vi "test.vi"() -> ()   [LabVIEW 2020]
uses:
  DSF Core.lvlibp/Typedefs/DSF Engine Framework Configuration.ctl
  DSF Core.lvlibp/Typedefs/DSF Engine Plugin Configuration.ctl
  DSF Core.lvlibp/Typedefs/Core Plugin Configuration.ctl
  DSF Core.lvlibp/Typedefs/DSF Timing Info.ctl
  DSF Core.lvlibp/Typedefs/DSF Settings Info.ctl
  DSF Core.lvlibp/Typedefs/DSF Engine Plugin Thread Configuration.ctl
  DSF Core.lvlibp/Typedefs/Core Thread Configuration.ctl
  DSF Core.lvlibp/Typedefs/DSF Engine Transfer Group Configuration.ctl
  DSF Core.lvlibp/Typedefs/Core Group Configuration.ctl
  DSF Core.lvlibp/Typedefs/DSF Direction.ctl
  DSF Core.lvlibp/Typedefs/DSF Timeout Behavior.ctl
  DSF Core.lvlibp/Typedefs/DSF Engine Transfer Configuration.ctl
  DSF Core.lvlibp/Typedefs/Core Transfer Configuration.ctl
  DSF Core.lvlibp/Typedefs/DSF Engine Channel Configuration.ctl
  DSF Core.lvlibp/Typedefs/Core Channel Configuration.ctl
  DSF Core.lvlibp/Typedefs/DSF Data Type.ctl
  niveristand-data-sharing-framework-custom-device/Source/Core/Built/Configuration API/Component/Default Buffer Converter/Default Buffer Converter Transfer Settings.ctl
  DSF Core.lvlibp/Typedefs/DSF Byte Order.ctl
  Types/Tx Configuration.ctl
  Built/Plugins/Windows/Components/UDP.lvlibp/Configuration/Thread/Thread Settings.ctl
  niveristand-data-sharing-framework-custom-device/Source/Core/Built/Configuration API/DSF Configuration API.lvlib
  DSF Core.lvlibp
  DSF Core.lvlibp/Classes/Configuration/Core/Plugin/Plugin Configuration.lvclass
  DSF Core.lvlibp/Classes/Configuration/Core/Channel/Channel Configuration.lvclass
  DSF Core.lvlibp/Classes/Configuration/Core/Group/Group Configuration.lvclass
  DSF Core.lvlibp/Classes/Configuration/Core/Thread/Thread Configuration.lvclass
  DSF UDP Configuration API.lvlib
  Built/Plugins/Windows/Components/UDP.lvlibp/Configuration/Thread/UDP Thread Configuration.lvclass
  DSF Core.lvlibp/Classes/Configuration/Core/Transfer/Transfer Configuration.lvclass
panel:
  out "framework out":T1
  out "error out":errorcluster
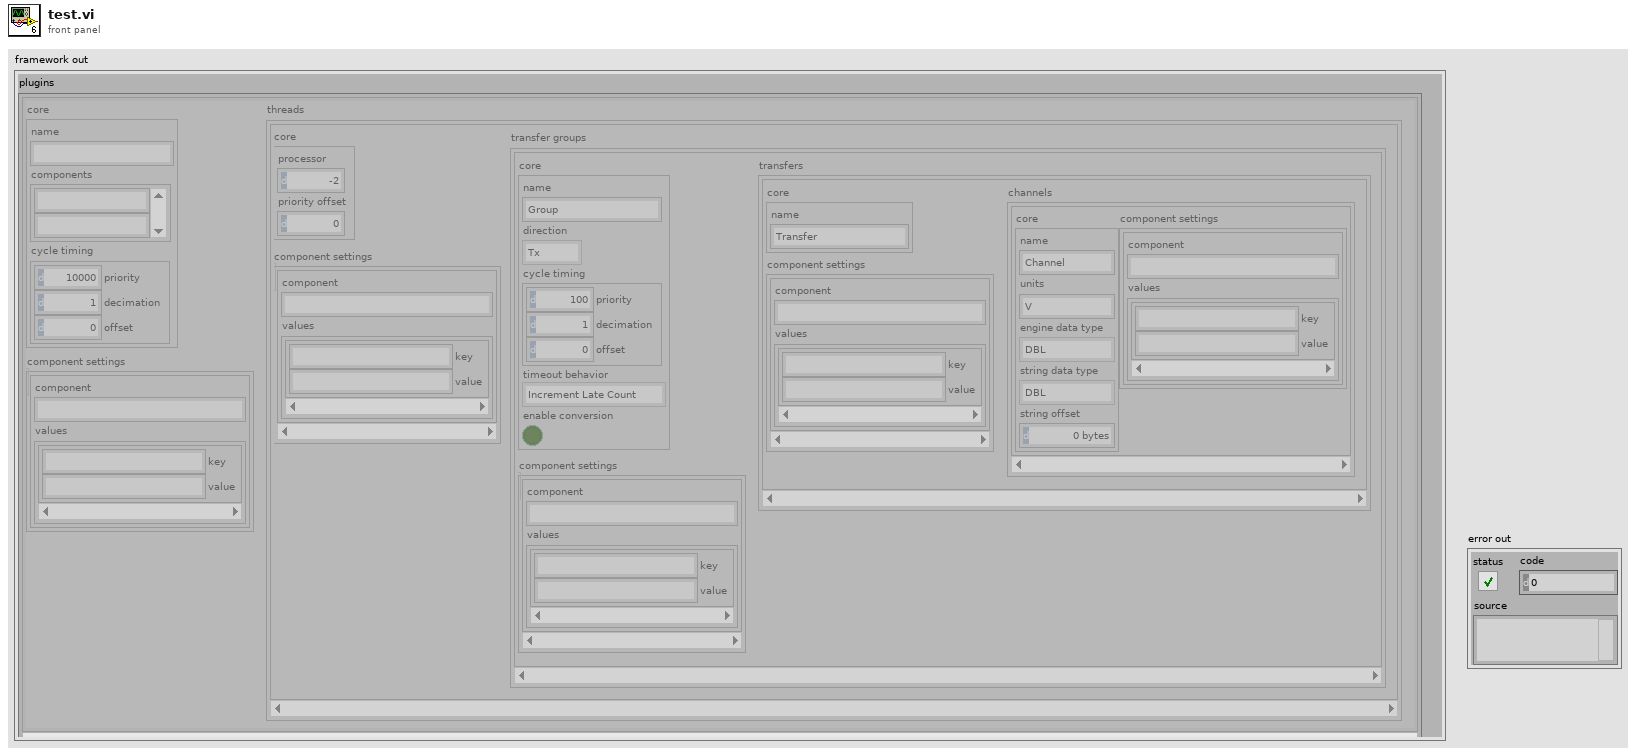
[diagram p1: front panel]
types:
  T1 = typedef "DSF Core.lvlibp/DSF Engine Framework Configuration.ctl" = cluster{"plugins":T2[]}
  T2 = typedef "DSF Core.lvlibp/DSF Engine Plugin Configuration.ctl" = cluster{"core":T3, "component settings":T5[], "threads":T6[]}
  T3 = typedef "DSF Core.lvlibp/Plugin Configuration.lvclass/Core Plugin Configuration.ctl" = cluster{"name":string, "components":string[], "cycle timing":T4}
  T4 = typedef "DSF Core.lvlibp/DSF Timing Info.ctl" = cluster{"priority":u64, "decimation":u64, "offset":u64}
  T5 = typedef "DSF Core.lvlibp/DSF Settings Info.ctl" = cluster{"component":string, "values":cluster{"key":string, "value":string}[]}
  T6 = typedef "DSF Core.lvlibp/DSF Engine Plugin Thread Configuration.ctl" = cluster{"core":T7, "component settings":T5[], "transfer groups":T8[]}
  T7 = typedef "DSF Core.lvlibp/Thread Configuration.lvclass/Core Thread Configuration.ctl" = cluster{"processor":i32, "priority offset":i16}
  T8 = typedef "DSF Core.lvlibp/DSF Engine Transfer Group Configuration.ctl" = cluster{"core":T9, "component settings":T5[], "transfers":T12[]}
  T9 = typedef "DSF Core.lvlibp/Group Configuration.lvclass/Core Group Configuration.ctl" = cluster{"name":string, "direction":T10, "cycle timing":T4, "timeout behavior":T11, "enable conversion":bool}
  T10 = typedef "DSF Core.lvlibp/DSF Direction.ctl" = enum8{"Tx", "Rx"}
  T11 = typedef "DSF Core.lvlibp/DSF Timeout Behavior.ctl" = enum8{"Increment Late Count", "Throw Error"}
  T12 = typedef "DSF Core.lvlibp/DSF Engine Transfer Configuration.ctl" = cluster{"core":T13, "component settings":T5[], "channels":T14[]}
  T13 = typedef "DSF Core.lvlibp/Transfer Configuration.lvclass/Core Transfer Configuration.ctl" = cluster{"name":string}
  T14 = typedef "DSF Core.lvlibp/DSF Engine Channel Configuration.ctl" = cluster{"core":T15, "component settings":T5[]}
  T15 = typedef "DSF Core.lvlibp/Channel Configuration.lvclass/Core Channel Configuration.ctl" = cluster{"name":string, "units":string, "engine data type":T16, "string data type":T16, "string offset":u64}
  T16 = typedef "DSF Core.lvlibp/DSF Data Type.ctl" = enum8{"Bool", "SGL", "DBL", "I8", "I16", "I32", "I64", "U8", "U16", "U32", "U64"}
  T17 = typedef "UDP.lvlibp/UDP Thread Configuration.lvclass/Thread Settings.ctl" = cluster{"local port":u16, "local address":u32}
  T18 = typedef "DSF UDP Configuration API.lvlib/Tx Configuration.ctl" = cluster{"destination address":string, "destination port":u16}
  T19 = typedef "DSF Configuration API.lvlib/Default Buffer Converter Transfer Settings.ctl" = cluster{"byte order":T20}
  T20 = typedef "DSF Core.lvlibp/DSF Byte Order.ctl" = enum8{"big-endian", "little-endian"}
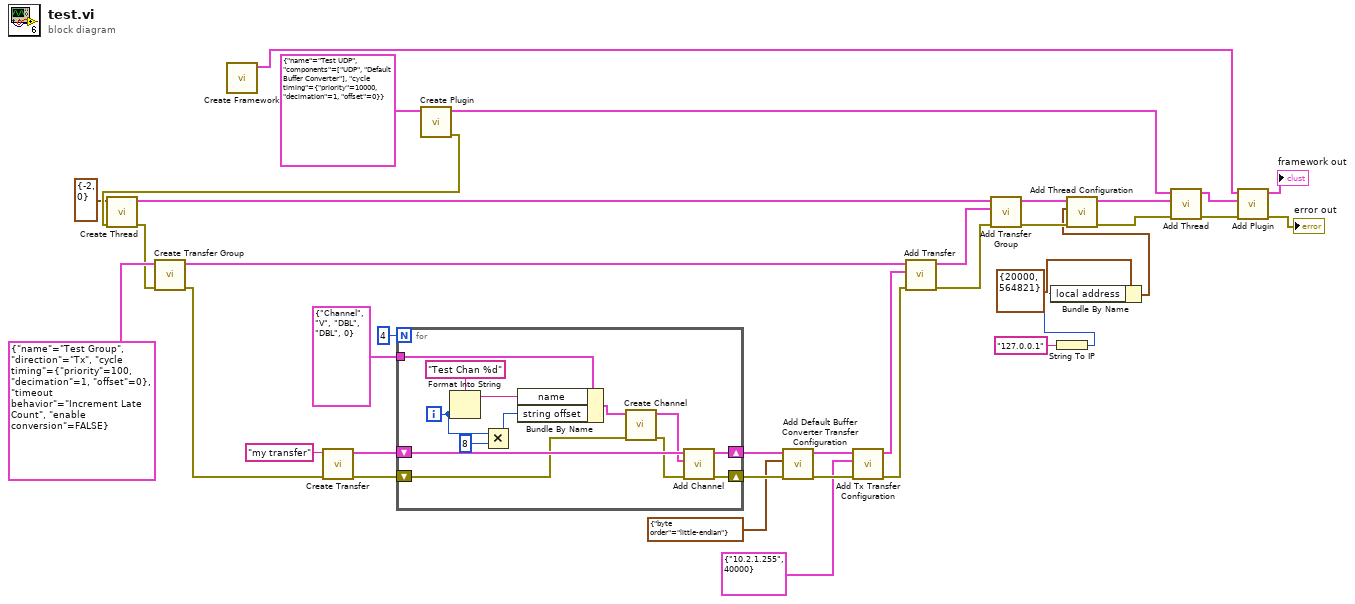
[diagram p0: block diagram]
diagram:
  n1 = call "Create Framework.vi"() -> ("framework"=w22:T1)  [unwired: 11 in]
  n2 = call "Create Plugin.vi"("configuration"=T3 {"name"="Test UDP", "components"=["UDP", "Default Buffer Converter"], "cycle timing"={"priority"=10000, "decimation"=1, "offset"=0}}) -> ("error out"=w25:errorcluster, "plugin"=w26:T2)  [unwired: 9 in]
  n3 = call "Create Thread.vi"("error in"=w25, "configuration"=T7 {"processor"=-2, "priority offset"=0}) -> ("error out"=w27:errorcluster, "thread"=w28:T6)  [unwired: 8 in]
  n4 = call "Create Transfer Group.vi"("error in"=w27, "configuration"=T9 {"name"="Test Group", "direction"=enum."Tx", "cycle timing"={"priority"=100, "decimation"=1, "offset"=0}, "timeout behavior"=enum."Increment Late Count", "enable conversion"=FALSE}) -> ("error out"=w31:errorcluster, "transfer group"=w29:T8)  [unwired: 8 in]
  n5 = call "Create Transfer.vi"("error in"=w31, "name"="my transfer") -> ("error out"=w32:errorcluster, "transfer"=w33:T12)  [unwired: 8 in]
  n6 = for {
    N: 4 -> [_]
    tunnel: T15 {"name"="Channel", "units"="V", "engine data type"=enum."DBL", "string data type"=enum."DBL", "string offset"=0} ("configuration") -> [w49]
    shift-right: [w45] -> w17
    shift-left: w33 -> [w46]
    shift-right: [w42] -> w18
    shift-left: w32 -> [w44]
    i -> [w39]
    n7 = Format Into String(format string="Test Chan %d", w39) -> (resulting string=w48:string)  [unwired: 2 in, 1 out]
    n8 = Multiply(x=w39, y=8) -> (x*y=w40:i32)
    n9 = Bundle By Name(cluster=w49, "name"=w48, "string offset"=w40) -> (w47:T15)
    n10 = call "Create Channel.vi"("error in"=w44, "configuration"=w47) -> ("error out"=w43:errorcluster, "channel"=w41:T14)  [unwired: 8 in]
    n11 = call "Add Channel.vi"("error in"=w43, "channel"=w41, "transfer"=w46) -> ("error out"=w42:errorcluster, "transfer out"=w45:T12)  [unwired: 7 in]
  }
  n12 = call "Add Default Buffer Converter Transfer Configuration.vi"("error in"=w18, "transfer settings"=T19 {"byte order"=enum."little-endian"}, "transfer"=w17) -> ("error out"=w15:errorcluster, "transfer out"=w14:T12)  [unwired: 7 in]
  n13 = call "Add Tx Transfer Configuration.vi"("error in"=w15, "configuration"=T18 {"destination address"="10.2.1.255", "destination port"=40000}, "transfer"=w14) -> ("error out"=w11:errorcluster, "transfer out"=w12:T12)  [unwired: 7 in]
  n14 = call "Add Transfer.vi"("error in"=w11, "transfer"=w12, "transfer group"=w29) -> ("error out"=w9:errorcluster, "transfer group out"=w10:T8)  [unwired: 7 in]
  n15 = call "Add Transfer Group.vi"("error in"=w9, "transfer group"=w10, "thread"=w28) -> ("error out"=w7:errorcluster, "thread out"=w8:T6)  [unwired: 7 in]
  n16 = String To IP(1:"127.0.0.1" ("name")) -> (0:w2:u32)
  n17 = Bundle By Name(cluster=T17 {"local port"=20000, "local address"=564821} ("configuration"), "local address"=w2) -> (w1:T17)
  n18 = call "Add Thread Configuration.vi"("error in"=w7, "configuration"=w1, "thread"=w8) -> ("error out"=w6:errorcluster, "thread out"=w5:T6)  [unwired: 7 in]
  n19 = call "Add Thread.vi"("error in"=w6, "thread"=w5, "plugin"=w26) -> ("error out"=w23:errorcluster, "plugin out"=w21:T2)  [unwired: 7 in]
  n20 = call "Add Plugin.vi"("error in"=w23, "plugin"=w21, "framework"=w22) -> ("error out"=→"error out":errorcluster, "framework out"=→"framework out":T1)  [unwired: 7 in]
